vi "Get Channels.vi"(8 "error in (no error)":errorcluster, 11 "Group Config in":refnum<class "Group Config.lvclass">) -> (0 "error out":errorcluster, 2 "Channels":refnum<class "Channel Config.lvclass">[](array[class]), 3 "Group Config out":refnum<class "Group Config.lvclass">)   [LabVIEW 2020, in "Vecto.lvlib" / "Group Config.lvclass"]
uses:
  Group Config.lvclass
  Channel Config/Channel Config.lvclass
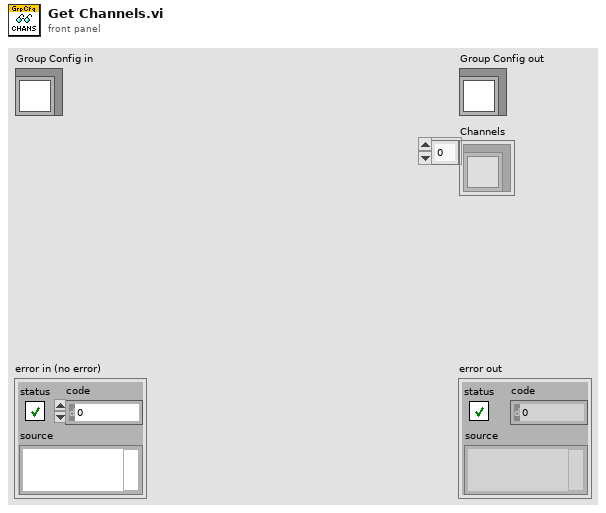
[diagram p1: front panel]
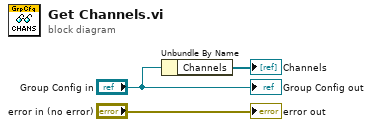
[diagram p0: block diagram]
diagram:
  n1 = Unbundle By Name("Group Config in") -> ("Channels"=→"Channels":refnum<class "Channel Config.lvclass">[])
  "error out" <- "error in (no error)"
  "Group Config out" <- "Group Config in"
